vi "LoadJSONVarIntoVM.vi"(8 "error in (no error)":errorcluster, 10 "JSON Variable Object":string, 11 "VariableManagerRef in":refnum<vi>) -> (0 "error out":errorcluster, 3 "VariableManagerRef out":refnum<vi>)   [LabVIEW 2013]
doc: "Takes a variable in JSON form and either updates the Variable Manager variable or creates a new one."
uses:
  VariableManagerCodes/VariableManager/VariableManager.lvclass
  <vilib>/regexp/Match Regular Expression.xnode
  VariableManagerCodes/API/VariableManagerAPI.lvlib
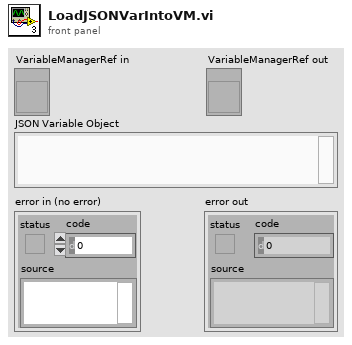
[diagram p1: front panel]
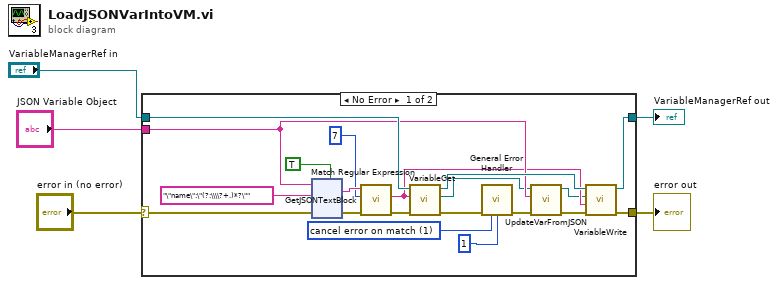
[diagram p0: block diagram]
diagram:
  n1 = case shown="No Error" "error in (no error)" {
    selector: "error in (no error)" -> [w7 w141]
    tunnel: "VariableManagerRef in" -> [w22 w140]
    tunnel: [w21 w140] -> w4
    tunnel: "JSON Variable Object" -> [w14 _]
    tunnel: [w8 w141] -> w2
    frame No Error {
      w17 = 1 items=["no exception", "cancel error on match", "set error on match"] ("[exception action] (none:0)")
      n2 = xnode "Match Regular Expression"("input string"=w14, "regular expression"="\"name\":\"(?:\\\\?+.)*?\"", "error in"=w7, "multiline? (F)"=TRUE) -> ("whole match"=w24:string, "error out"=w19:errorcluster)  [unwired: 2 in, 3 out]
      n3 = call "GetJSONTextBlock.vi"("error in (no error)"=w19, "Block Start Offset"=7, "String In"=w24) -> ("error out"=w18:errorcluster, "Matched Block Contents"=w11:string)  [unwired: 4 in, 3 out]
      n4 = call "VariableGet.vi"("error in (no error)"=w18, "VariableName"=w11, "VariableManagerRef in"=w22) -> ("error out"=w15:errorcluster, "Variable"=w12:refnum<class "Variable.lvclass">, "VariableManagerRef out"=w20:refnum<vi>)  [unwired: 6 in]
      n5 = call <vilib>:"General Error Handler.vi"("error in (no error)"=w15, "[exception action] (none:0)"=w17, "[exception code]"=1) -> ("error out"=w6:errorcluster)  [unwired: 8 in, 4 out]
      n6 = call "UpdateVarFromJSON.vi"("error in (no error)"=w6, "JSON Variable Object"=w14, "Variable.lvclass"=w12) -> ("error out"=w9:errorcluster, "reference out"=w10:refnum<class "Variable.lvclass">)  [unwired: 7 in]
      n7 = call "VariableWrite.vi"("error in (no error)"=w9, "OriginalName"=w11, "Variable"=w10, "VariableManagerRef in"=w20) -> ("error out"=w8:errorcluster, "VariableManagerRef out"=w21:refnum<vi>)  [unwired: 6 in]
    }
    frame Error {
    }
  }
  "VariableManagerRef out" <- w4
  "error out" <- w2
